vi "Write pointer.vi"(8 "error in (no error)":errorcluster, 10 "pointer":u64, 11 "POSIX Thread Object in":refnum<class "POSIX Thread Object.lvclass">) -> (0 "error out":errorcluster, 3 "POSIX Thread Object out":refnum<class "POSIX Thread Object.lvclass">)   [LabVIEW 2013, in "Linux RT IPC.lvlib" / "POSIX Threads.lvlib" / "POSIX Thread Object.lvclass"]
uses:
  POSIX Thread Object.lvclass
  POSIX Thread Object.lvclass/POSIX Thread Object.ctl
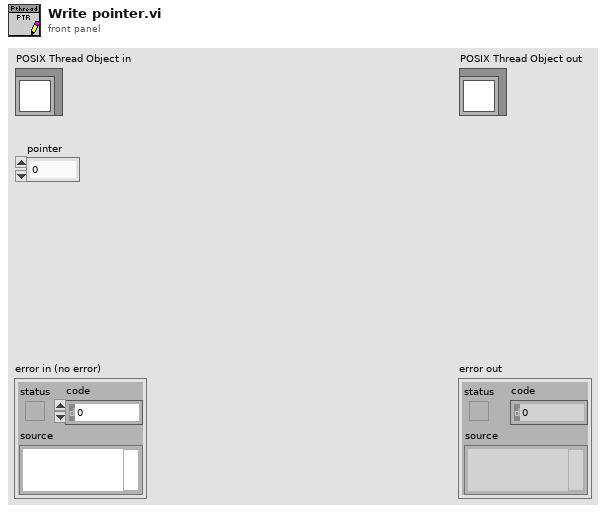
[diagram p1: front panel]
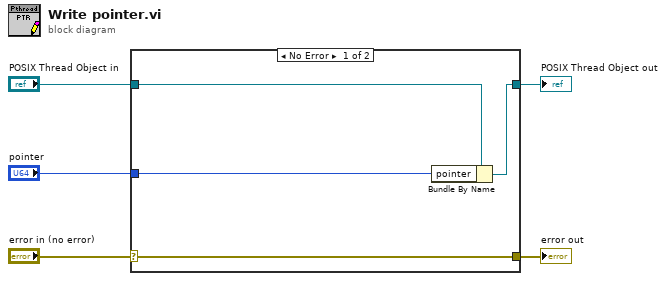
[diagram p0: block diagram]
diagram:
  n1 = case shown="No Error" "error in (no error)" {
    selector: "error in (no error)" -> [w9 w10]
    tunnel: [w9 w10] -> w4
    tunnel: [w7 w11] -> w2
    tunnel: "POSIX Thread Object in" -> [w8 w11]
    tunnel: "pointer" -> [w6 _]
    frame No Error {
      n2 = Bundle By Name(cluster=w8, "pointer"=w6) -> (w7:refnum<class "POSIX Thread Object.lvclass">)
    }
    frame Error {
    }
  }
  "error out" <- w4
  "POSIX Thread Object out" <- w2
